vi "ReadHBMFileSARAH.vi"(4 "error in (no error)":errorcluster, 6 "file path":path) -> (0 "error out":errorcluster, 2 "HBMWaveformsOut":waveform(dbl)[](graph))   [LabVIEW 2017]
panel:
  out "TailleYAvant":i32[](array[numeric])
  out "dtAvant":dbl[](array[numeric])
  out "dtApres":dbl[](array[numeric])
  out "TailleYApres":i32[](array[numeric])
  out "AllChannelsName":string[](array[string])
  out "ChannelNames 2":string[](array[string])
  out "size(s) 3":i32
  out "WaveformComputational":waveform(dbl)[](graph)
  out "ChannelUnit 2":string[](array[string])
  out "size(s) 2":i32
  out "Unit":string
  out "Name":string
  out "ChannelUnit":string[](array[string])
  out "ChannelNames":string[](array[string])
  out "Waveform Graph 2":waveform(dbl)(graph)
  out "WaveformHardware":waveform(dbl)[](graph)
  out "size(s)":i32
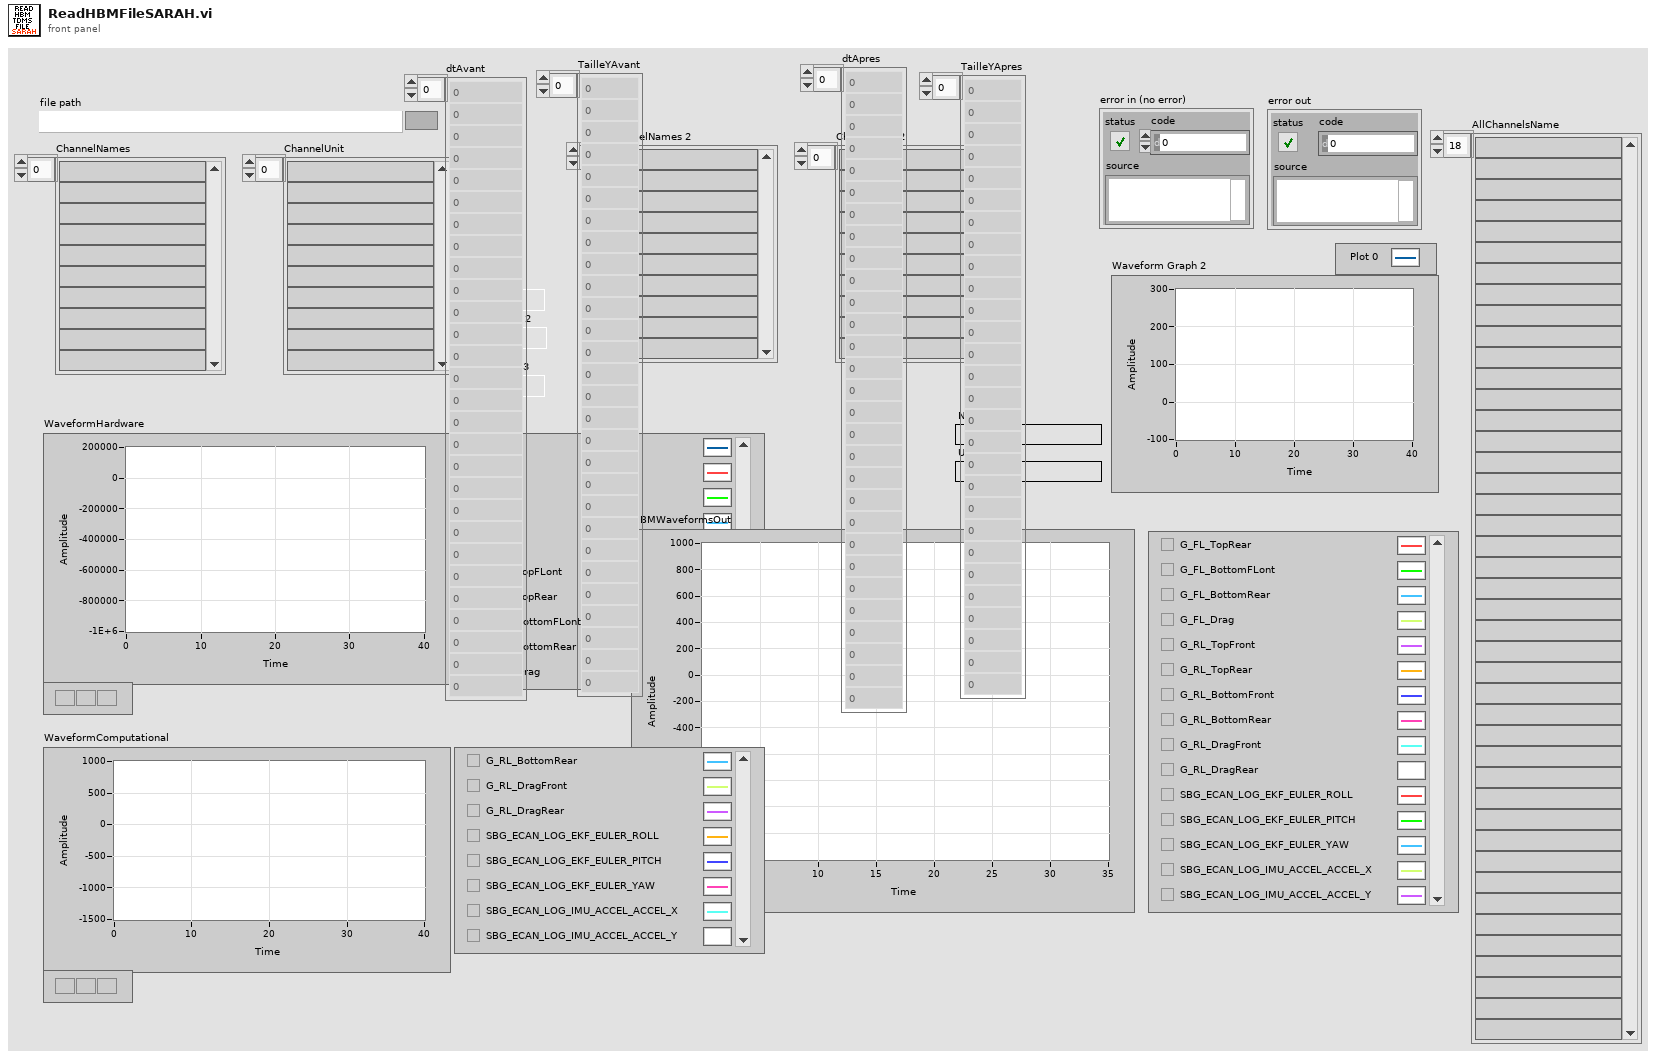
[diagram p1: front panel]
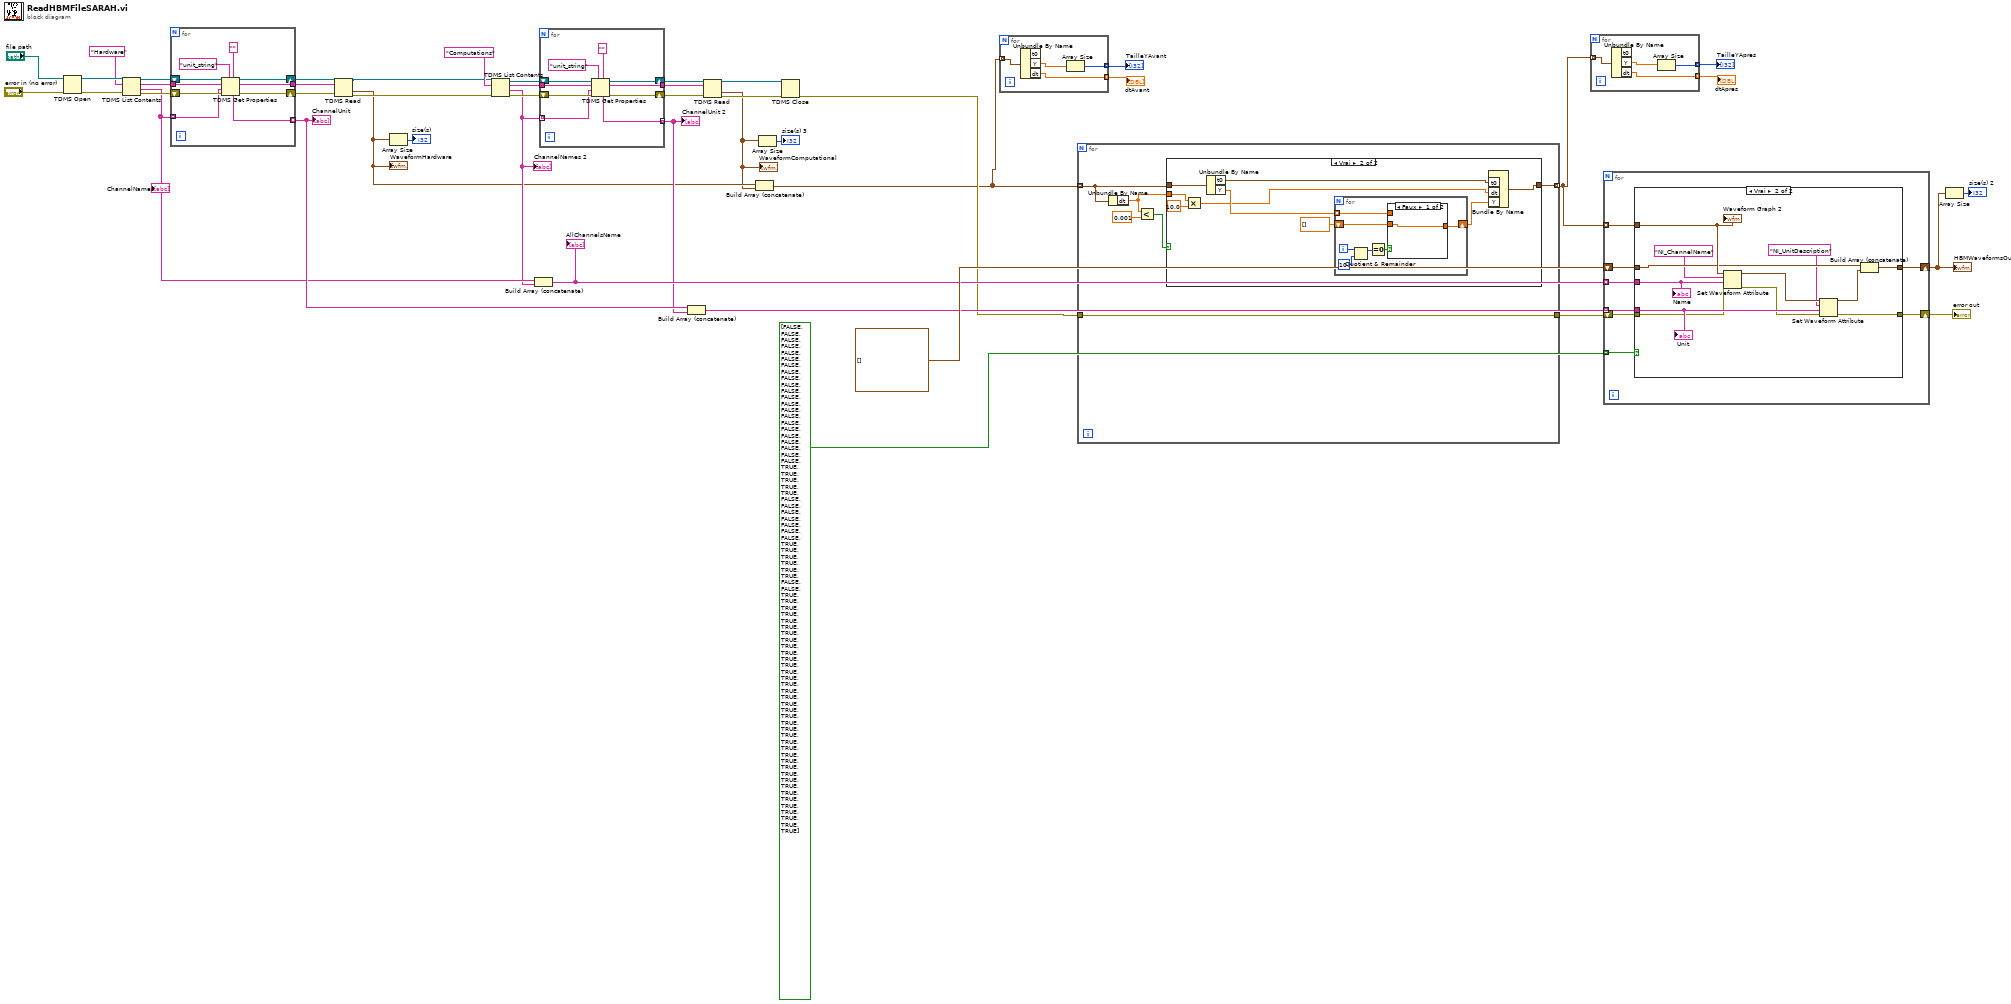
[diagram p0: block diagram]
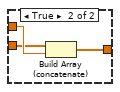
[diagram p3: hidden frame]
diagram:
  n1 = TDMS Open(8:"error in (no error)", 11:"file path") -> (0:w42:errorcluster, 3:w41:refnum<k34>)  [unwired: 5 in]
  n2 = TDMS List Contents(4:w42, 6:"Hardware" ("group name"), 7:w41) -> (0:w39:errorcluster, 1:w13:string[], 2:w37:string, 3:w40:refnum<k34>)
  "ChannelNames" <- w13
  n3 = for {
    tunnel: w37 -> [w51]
    shift-right: [w53] -> w36
    shift-left: w40 -> [w55]
    shift-right: [w52] -> w35
    shift-left: w39 -> [w54]
    tunnel: w13 -> [w48] mode=indexing
    tunnel: [w47] -> w15 mode=indexing
    tunnel: [w46] -> w34
    n4 = TDMS Get Properties(5:"" ("property name"), 7:"unit_string" ("property name"), 8:w54, 9:w48, 10:w51, 11:w55) -> (0:w52:errorcluster, 2:w46:string, 3:w53:refnum<k34>, 4:w47:string)  [unwired: 2 out]
  }
  "ChannelUnit" <- w15
  n5 = TDMS Read(0:w36, 5:w34, 11:w35) -> (4:w18:refnum<k34>, 10:w11:waveform(dbl)[], 15:w19:errorcluster)  [unwired: 5 in, 3 out]
  "WaveformHardware" <- w11
  n6 = Array Size(array=w11) -> (size(s)=→"size(s)":i32)
  n7 = TDMS List Contents(4:w19, 6:"Computations" ("group name"), 7:w18) -> (0:w24:errorcluster, 1:w12:string[], 2:w26:string, 3:w23:refnum<k34>)
  "ChannelNames 2" <- w12
  n8 = Build Array (concatenate)(w13, w12) -> (w17:string[])
  "AllChannelsName" <- w17
  n9 = for {
    tunnel: w26 -> [w61]
    shift-right: [w63] -> w27
    shift-left: w23 -> [w65]
    shift-right: [w62] -> w28
    shift-left: w24 -> [w64]
    tunnel: w12 -> [w58] mode=indexing
    tunnel: [w57] -> w14 mode=indexing
    tunnel: [w56] -> w29
    n10 = TDMS Get Properties(5:"" ("property name"), 7:"unit_string" ("property name"), 8:w64, 9:w58, 10:w61, 11:w65) -> (0:w62:errorcluster, 2:w56:string, 3:w63:refnum<k34>, 4:w57:string)  [unwired: 2 out]
  }
  "ChannelUnit 2" <- w14
  n11 = Build Array (concatenate)(w15, w14) -> (w16:string[])
  n12 = TDMS Read(0:w27, 5:w29, 11:w28) -> (4:w21:refnum<k34>, 10:w10:waveform(dbl)[], 15:w20:errorcluster)  [unwired: 5 in, 3 out]
  "WaveformComputational" <- w10
  n13 = Build Array (concatenate)(w11, w10) -> (w1:waveform(dbl)[])
  n14 = Array Size(array=w10) -> (size(s)=→"size(s) 3":i32)
  n15 = TDMS Close(8:w20, 11:w21) -> (0:w8:errorcluster)  [unwired: 1 out]
  n16 = for {
    tunnel: w1 -> [w69] mode=indexing
    tunnel: [w67] -> w2 mode=indexing
    tunnel: [w66] -> w3 mode=indexing
    n17 = Unbundle By Name(w69) -> ("Y"=w68:dbl[], "dt"=w66:dbl)  [unwired: 1 out]
    n18 = Array Size(array=w68) -> (size(s)=w67:i32)
  }
  "TailleYAvant" <- w2
  "dtAvant" <- w3
  n19 = for {
    tunnel: w1 -> [w74] mode=indexing
    tunnel: [w73] -> w6 mode=indexing
    tunnel: w8 -> [w71]
    tunnel: [w71] -> w7
    n20 = Unbundle By Name(w74) -> ("dt"=w72:dbl)
    n21 = Less?(x=w72, y=0.001) -> (x < y?=w70:bool)
    n22 = case shown="Vrai" w70 {
      tunnel: w74 -> [w76 w83]
      tunnel: [w76 w77] -> w73
      tunnel: w72 -> [_ w84]
      frame False {
      }
      frame True {
        n23 = Multiply(x=w84, y=10.0) -> (x*y=w79:dbl)
        n24 = Unbundle By Name(w83) -> ("t0"=w80:timestamp, "Y"=w82:dbl[])
        n25 = for {
          tunnel: w82 -> [w89] mode=indexing
          shift-right: [w88] -> w78
          shift-left: dbl[] [] -> [w87]
          i -> [w92]
          n26 = Quotient & Remainder(x=w92, y=10) -> (x-y*floor(x/y)=w90:i32)  [unwired: 1 out]
          n27 = Equal To 0?(x=w90) -> (x = 0?=w86:bool)
          n28 = case shown="Faux" w86 {
            tunnel: w89 -> [_ w96]
            tunnel: [w93 w95] -> w88
            tunnel: w87 -> [w93 w94]
            frame False {
            }
            frame True {
              n29 = Build Array (concatenate)(w94, w96) -> (w95:dbl[])
            }
          }
        }
        n30 = Bundle By Name("t0"=w80, "dt"=w79, "Y"=w78) -> (w77:waveform(dbl))  [unwired: 1 in]
      }
    }
  }
  n31 = for {
    tunnel: w6 -> [w100] mode=indexing
    tunnel: [w98] -> w5 mode=indexing
    tunnel: [w97] -> w4 mode=indexing
    n32 = Unbundle By Name(w100) -> ("Y"=w99:dbl[], "dt"=w97:dbl)  [unwired: 1 out]
    n33 = Array Size(array=w99) -> (size(s)=w98:i32)
  }
  "TailleYApres" <- w5
  "dtApres" <- w4
  n34 = for {
    tunnel: w6 -> [w108] mode=indexing
    tunnel: w17 -> [w105] mode=indexing
    tunnel: w16 -> [w107] mode=indexing
    shift-right: [w104] -> w30
    shift-left: waveform(dbl)[] [] -> [w103]
    shift-right: [w106] -> w33
    shift-left: w7 -> [w102]
    tunnel: bool[] [FALSE, FALSE, FALSE, FALSE, FALSE, FALSE, FALSE, FALSE, FALSE, FALSE, FALSE, FALSE, FALSE, FALSE, FALSE, FALSE, FALSE, FALSE, FALSE, FALSE, FALSE, FALSE, TRUE, TRUE, TRUE, TRUE, TRUE, FALSE, FALSE, FALSE, FALSE, FALSE, FALSE, FALSE, TRUE, TRUE, TRUE, TRUE, TRUE, TRUE, FALSE, FALSE, TRUE, TRUE, TRUE, TRUE, TRUE, TRUE, TRUE, TRUE, TRUE, TRUE, TRUE, TRUE, TRUE, TRUE, TRUE, TRUE, TRUE, TRUE, TRUE, TRUE, TRUE, TRUE, TRUE, TRUE, TRUE, TRUE, TRUE, TRUE, TRUE, TRUE, TRUE, TRUE, TRUE, TRUE, TRUE, TRUE, TRUE, TRUE] ("Tableau") -> [w101] mode=indexing
    n35 = case shown="Vrai" w101 {
      tunnel: w108 -> [_ w122]
      tunnel: w107 -> [_ w121]
      tunnel: [w109 w120] -> w106
      tunnel: w105 -> [_ w119]
      tunnel: [w110 w118] -> w104
      tunnel: w103 -> [w110 w117]
      tunnel: w102 -> [w109 w116]
      frame False {
      }
      frame True {
        n36 = Set Waveform Attribute(4:w116, 5:w119, 6:"NI_ChannelName" ("name"), 7:w122) -> (0:w115:errorcluster, 3:w114:waveform(dbl))  [unwired: 1 out]
        n37 = Set Waveform Attribute(4:w115, 5:w121, 6:"NI_UnitDescription" ("name"), 7:w114) -> (0:w120:errorcluster, 3:w111:waveform(dbl))  [unwired: 1 out]
        n38 = Build Array (concatenate)(w117, w111) -> (w118:waveform(dbl)[])
        "Waveform Graph 2" <- w122
        "Name" <- w119
        "Unit" <- w121
      }
    }
  }
  "HBMWaveformsOut" <- w30
  "error out" <- w33
  n39 = Array Size(array=w30) -> (size(s)=→"size(s) 2":i32)
